vi "Find_Unique_Filename.vi"(0 "Path In":path, 1 "Max Length (31)":i32=31) -> (3 "Unique Path Out":path)   [LabVIEW 2010]
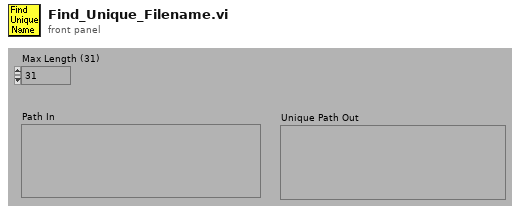
[diagram p1: front panel]
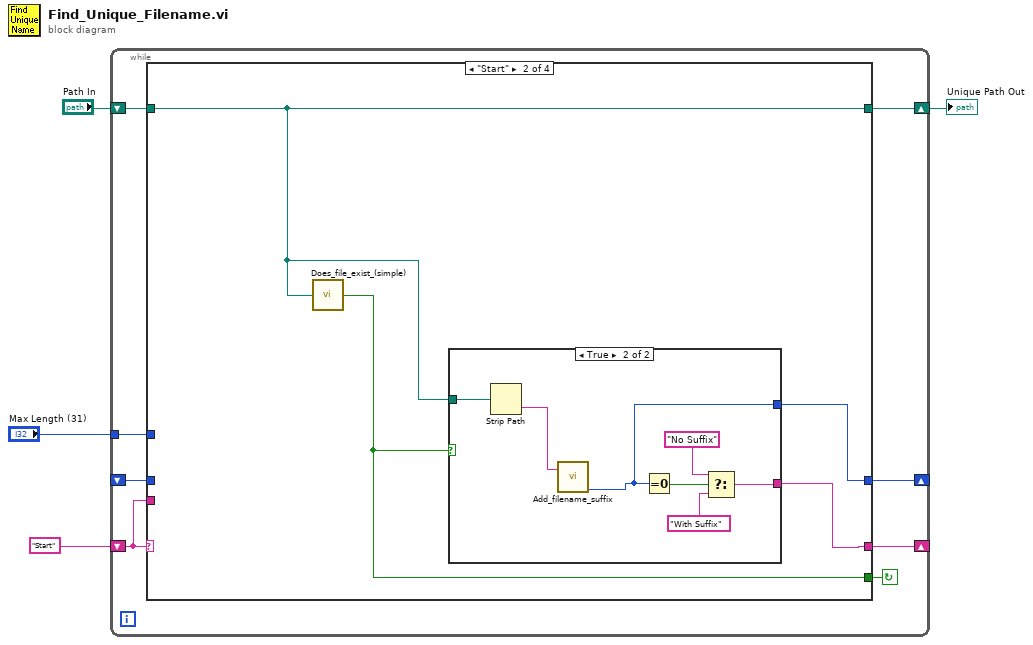
[diagram p0: block diagram]
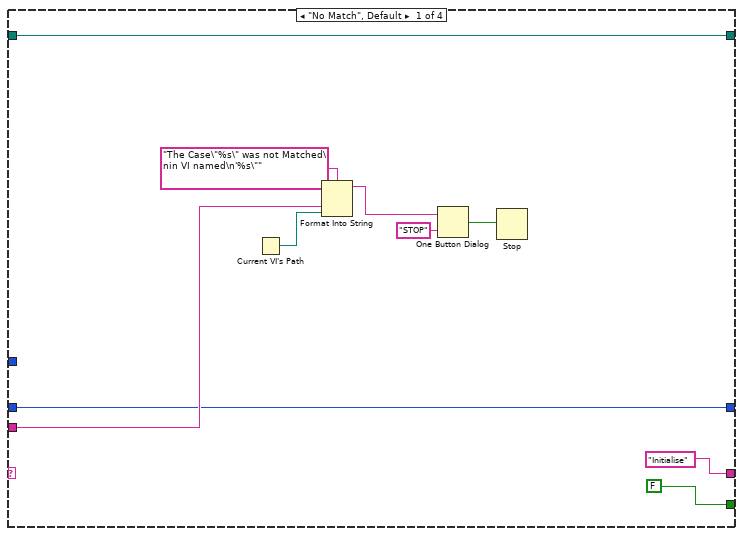
[diagram p2: hidden frame]
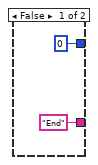
[diagram p3: hidden frame]
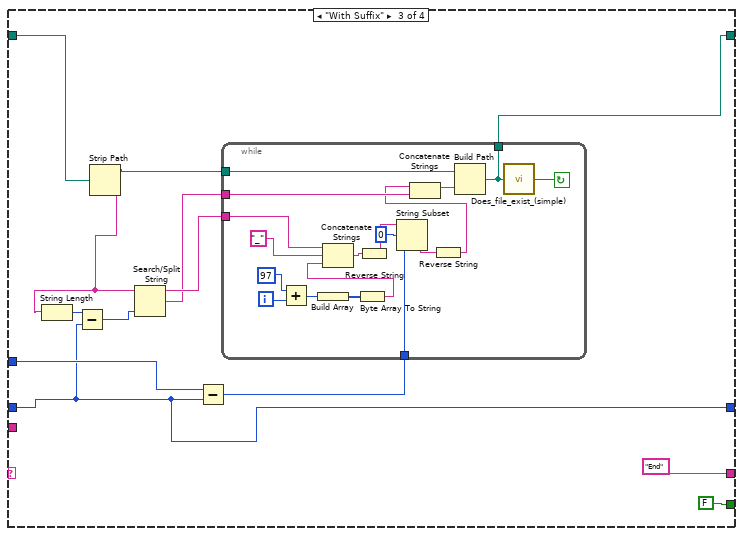
[diagram p4: hidden frame]
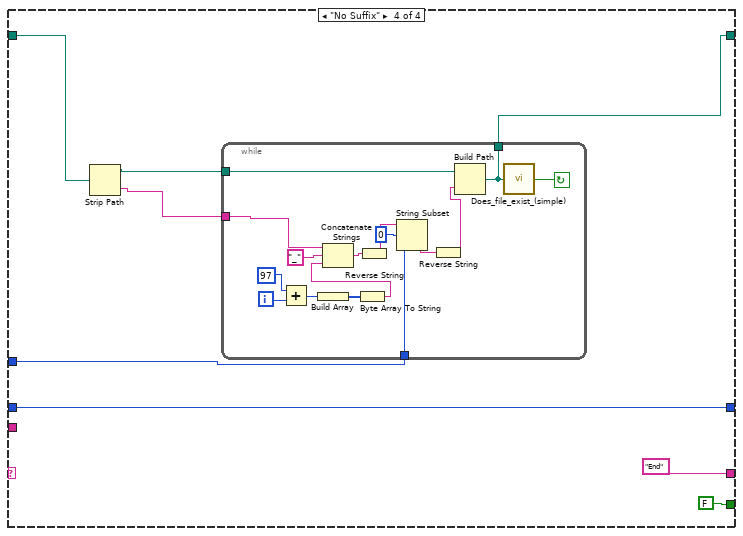
[diagram p5: hidden frame]
diagram:
  n1 = while {
    shift-left: "Start" -> [w10]
    shift-right: [w11] -> _
    shift-right: [w8] -> w2
    shift-left: "Path In" -> [w9]
    tunnel: "Max Length (31)" -> [w7]
    shift-right: [w6] -> _
    shift-left: _ -> [w5]
    stop <- w12 continue-if-true
    n2 = case shown="\"Start\"" w10 {
      tunnel: [FALSE w25 FALSE FALSE] -> w12
      tunnel: ["Initialise" w26 "End" "End"] -> w11
      tunnel: w10 -> [w17 _ _ _]
      tunnel: w9 -> [w14 w24 w41 w71]
      tunnel: [w14 w24 w40 w70] -> w8
      tunnel: w7 -> [_ _ w43 w68]
      tunnel: [w13 w23 w36 w67] -> w6
      tunnel: w5 -> [w13 _ w36 w67]
      frame "No Match", Default {
        n3 = Current VI's Path() -> (path=w16:path)
        n4 = Format Into String(format string="The Case\"%s\" was not Matched\nin VI named\n'%s\"" ("Format String"), w17, w16) -> (resulting string=w20:string)  [unwired: 2 in, 1 out]
        n5 = One Button Dialog(message=w20, button name ("OK")="STOP") -> (true=w18:bool)
        n6 = Stop(stop? (T)=w18) -> ()
      }
      frame "Start" {
        n7 = call "Does_file_exist_(simple).vi"("Pathname"=w24) -> ("exists?"=w25:bool)
        n8 = case shown="True" w25 {
          tunnel: ["End" w34] -> w26
          tunnel: w24 -> [_ w31]
          tunnel: [0 ("Extension length") w29] -> w23
          frame False {
          }
          frame True {
            n9 = Strip Path(path=w31) -> (name=w30:string)  [unwired: 1 out]
            n10 = call "Add_filename_suffix.vi"("Filename"=w30) -> ("Extension length"=w29:i32)  [unwired: 1 in, 3 out]
            n11 = Equal To 0?(x=w29) -> (x = 0?=w35:bool)
            n12 = Select(t="No Suffix", s=w35, f="With Suffix") -> (s? t:f=w34:string)
          }
        }
      }
      frame "With Suffix" {
        n13 = Strip Path(path=w41) -> (stripped path=w46:path, name=w45:string)
        n14 = String Length(string=w45) -> (length=w44:i32)
        n15 = Subtract(x=w44, y=w36) -> (x-y=w39:i32)
        n16 = Search/Split String(string=w45, offset (0)=w39) -> (substring before match=w38:string, match + rest of string=w37:string)  [unwired: 2 out]
        n17 = Subtract(x=w43, y=w36) -> (x-y=w42:i32)
        n18 = while {
          tunnel: w38 -> [w66]
          tunnel: w42 -> [w65]
          tunnel: w46 -> [w64]
          tunnel: w37 -> [w63]
          tunnel: [w51] -> w40
          i -> [w53]
          stop <- w52 continue-if-true
          n19 = Add(x=97, y=w53) -> (x+y=w61:i32)
          n20 = Build Array(w61) -> (w62:i32[])
          n21 = Byte Array To String(unsigned byte array=w62) -> (string=w50:string)
          n22 = Concatenate Strings(w66, "_" ("string"), w50) -> (w58:string)
          n23 = Reverse String(1:w58) -> (0:w59:string)
          n24 = String Subset(string=w59, offset (0)=0, length (rest)=w65) -> (substring=w57:string)
          n25 = Reverse String(1:w57) -> (0:w55:string)
          n26 = Concatenate Strings(w55, w63) -> (w54:string)
          n27 = Build Path(base path=w64, name or relative path=w54) -> (appended path=w51:path)
          n28 = call "Does_file_exist_(simple).vi"("Pathname"=w51) -> ("exists?"=w52:bool)
        }
      }
      frame "No Suffix" {
        n29 = Strip Path(path=w71) -> (stripped path=w72:path, name=w69:string)
        n30 = while {
          tunnel: w69 -> [w90]
          tunnel: w68 -> [w89]
          tunnel: w72 -> [w88]
          tunnel: [w78] -> w70
          i -> [w80]
          stop <- w79 continue-if-true
          n31 = Add(x=97, y=w80) -> (x+y=w86:i32)
          n32 = Build Array(w86) -> (w87:i32[])
          n33 = Byte Array To String(unsigned byte array=w87) -> (string=w76:string)
          n34 = Concatenate Strings(w90, "_" ("string"), w76) -> (w83:string)
          n35 = Reverse String(1:w83) -> (0:w84:string)
          n36 = String Subset(string=w84, offset (0)=0, length (rest)=w89) -> (substring=w82:string)
          n37 = Reverse String(1:w82) -> (0:w77:string)
          n38 = Build Path(base path=w88, name or relative path=w77) -> (appended path=w78:path)
          n39 = call "Does_file_exist_(simple).vi"("Pathname"=w78) -> ("exists?"=w79:bool)
        }
      }
    }
  }
  "Unique Path Out" <- w2
